vi "Set Condition for Waveform Stream.vi"   [LabVIEW 2020, in "NI_VS Waveform Streaming Interface.lvlib"]
doc: "Defines the condition under which NI VeriStand streams waveform data to a host computer."
uses:
  <vilib>/NI VeriStand/Execution/WaveformStreaming/NI_VS Waveform Streaming Interface.lvlib
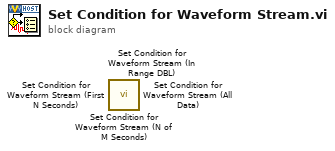
[diagram p0: block diagram]
diagram:
  n1 = call <vilib>:"Set Condition for Waveform Stream (N of M Seconds).vi"() -> ()  [unwired: 10 in, 2 out]
  n2 = call <vilib>:"Set Condition for Waveform Stream (In Range DBL).vi"() -> ()  [unwired: 10 in, 2 out]
  n3 = call <vilib>:"Set Condition for Waveform Stream (First N Seconds).vi"() -> ()  [unwired: 10 in, 2 out]
  n4 = call <vilib>:"Set Condition for Waveform Stream (All Data).vi"() -> ()  [unwired: 10 in, 2 out]
